vi "odor config arr to active odor set (sub-vi).vi"(10 "odor descriptions":T2) -> (2 "active odor chanel set":set{T1}(c389))   [LabVIEW 2021]
uses:
  type-defs/odor description array (type def).ctl
  type-defs/odor info cluster (type def).ctl
  type-defs/odor selection (type def).ctl
  type-defs/odor color (type def).ctl
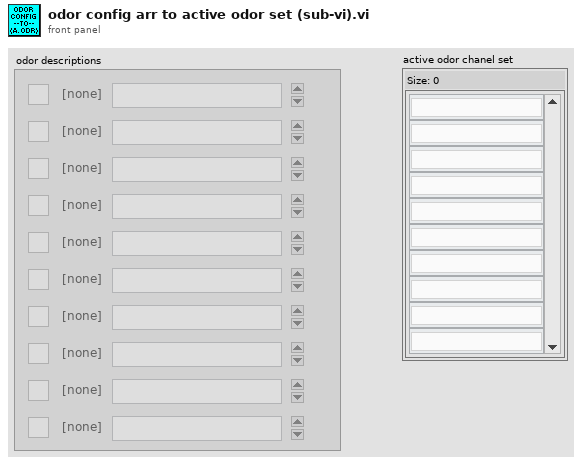
[diagram p1: front panel]
types:
  T1 = typedef "odor selection (type def).ctl" = enum16{"[none]", "odor 1", "odor 2", "odor 3", "odor 4", "odor 5", "odor 6", "odor 7", "odor 8", "odor 9", "odor 10"}
  T2 = typedef "odor description array (type def).ctl" = T3[]
  T3 = typedef "odor info cluster (type def).ctl" = cluster{"odor channel":T1, "odor description":string, "odor color":T4, "odor channel active":bool}
  T4 = typedef "odor color (type def).ctl" = u16
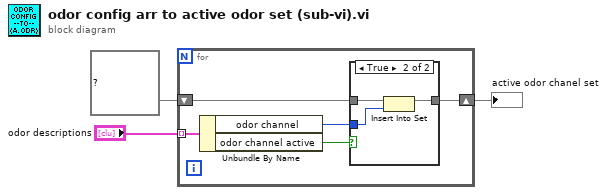
[diagram p0: block diagram]
diagram:
  n1 = for {
    tunnel: "odor descriptions" -> [w8] mode=indexing
    shift-right: [w4] -> w1
    shift-left: set{T1} {} ("odor channel") -> [w6]
    n2 = Unbundle By Name(w8) -> ("odor channel"=w5:T1, "odor channel active"=w7:bool)
    n3 = case shown="True" w7 {
      tunnel: w6 -> [w9 w11]
      tunnel: w5 -> [_ w12]
      tunnel: [w9 w10] -> w4
      frame False {
      }
      frame True {
        n4 = Insert Into Set(10:w12, 11:w11) -> (3:w10:set{T1})  [unwired: 1 out]
      }
    }
  }
  "active odor chanel set" <- w1
